vi "Add or Configure Endpoint.vi"(8 "error in (no error)":errorcluster, 9 "Configuration Type":T1, 10 "Endpoint":string, 11 "Endpoint Config Section Ref in":T2 format="%.0x") -> (0 "error out":errorcluster, 3 "Endpoint Config Section Ref out":T2 format="%.0x")   [LabVIEW 2017, in "SLSC Switch Scripting.lvlib"]
uses:
  SLSC Switch Scripting.lvlib
  <vilib>/NI Veristand/Custom Device API/Custom Device Item Ref.ctl
  Endpoint Configuration Enum.ctl
  <vilib>/NI Veristand/Custom Device API/Set Item Property (String).vi
  <vilib>/NI VeriStand/Custom Device API/Custom Device API.lvlib
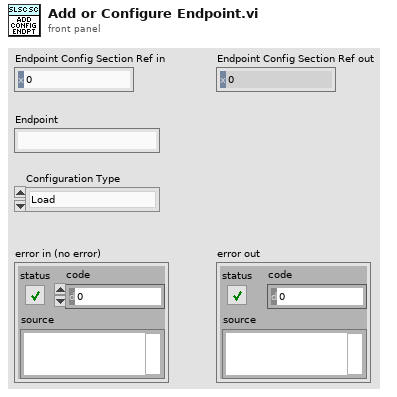
[diagram p1: front panel]
types:
  T1 = typedef "SLSC Switch Scripting.lvlib/Endpoint Configuration Enum.ctl" = enum16{"Load", "Source", "Configuration"}
  T2 = typedef "Custom Device API.lvlib/Custom Device Item Ref.ctl" = u64
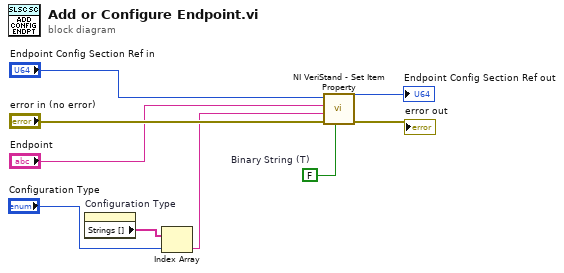
[diagram p0: block diagram]
diagram:
  w1 = FALSE  # Binary String (T)
  n1 = property on="Configuration Type" class="Enum (strict)"() -> ("Strings []"=w4:string[])  [unwired: 2 in, 2 out]
  n2 = Index Array(array=w4, index="Configuration Type") -> (element=w2:string)
  n3 = call-poly <vilib>:"NI VeriStand - Set Item Property.vi"("Binary String (T)"=w1, "error in (no error)"="error in (no error)", "Value"=w2, "Property Name"="Endpoint", "Item Ref in"="Endpoint Config Section Ref in") -> ("error out"=→"error out":errorcluster, "Item Ref out"=→"Endpoint Config Section Ref out":T2)  [unwired: 4 in, 1 out]
